vi "Create.vi"(7 "Direction":T1, 8 "error in (no error)":errorcluster, 9 "Custom Config Data":u8[](array[numeric]), 10 "Name":string, 11 "CIFTag in":refnum<class "CIF_NIChn_Fifo_Power.lvclass">) -> (0 "error out":errorcluster, 3 "CIFTag out":refnum<class "CIF_NIChn_Fifo_Power.lvclass">)   [LabVIEW 2021, in "CIF_NIChn_Fifo_Power.lvclass"]
uses:
  CIF_NIChn_Fifo_Power.lvclass
  CIF_NIChn_Fifo_Power.lvclass/CIF_NIChn_Fifo_Power.ctl
  CIFChannels/CIFChannels.lvclass
  CIFChannels/Typedef/Disconnect Behavior.ctl
  CIFChannels/Typedef/Channel State.ctl
  05c6e502-0377-480c-a15d-085597602460.vi
  c6f1aac1-fdda-4143-8087-f9e7d57e6170.vi
  D:/dev/Packages/Channel_Manager/src/CIF_NIChn/NIChn/CIF_NIChn.lvclass
  D:/dev/Packages/Channel_Manager/src/CIFChannels/CIFChannels.lvclass
  D:/dev/Packages/Channel_Manager/src/CIF_NIChn/FIFO_Power/CIF_NIChn_Fifo_Power.lvclass
  CIFChannels/Typedef/Direction.ctl
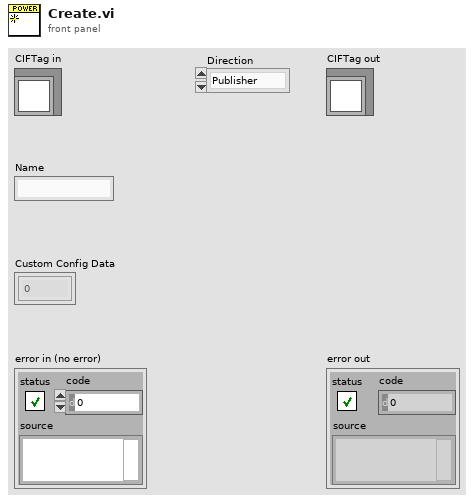
[diagram p1: front panel]
types:
  T1 = typedef "CIFChannels.lvclass/Direction.ctl" = enum16{"Publisher", "Subscriber"}
  T2 = typedef "CIFChannels.lvclass/Disconnect Behavior.ctl" = enum16{"Default value", "Last value", "Error with default"}
  T3 = typedef "CIFChannels.lvclass/Channel State.ctl" = enum16{"Creating", "Disconnected", "Connecting", "Connected", "Destroyed"}
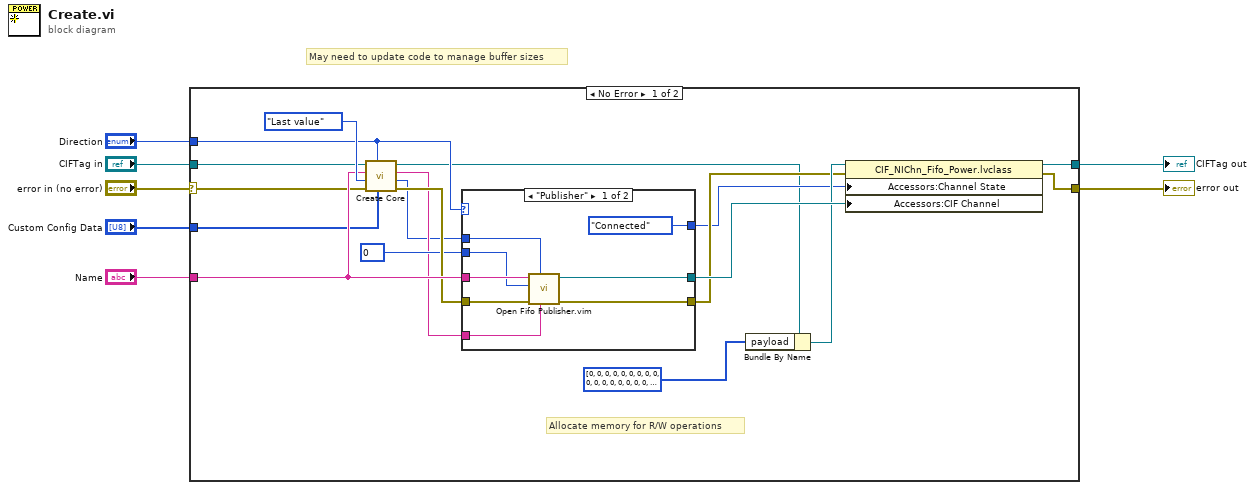
[diagram p0: block diagram]
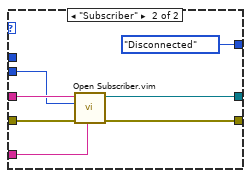
[diagram p2: hidden frame]
diagram:
  # "May need to update code to manage buffer sizes"
  n1 = case shown="No Error" "error in (no error)" {
    selector: "error in (no error)" -> [w9 w42]
    tunnel: [w8 w42] -> w6
    tunnel: [w19 w41] -> w4
    tunnel: "CIFTag in" -> [w10 w41]
    tunnel: "Name" -> [w24 _]
    tunnel: "Direction" -> [w18 _]
    tunnel: "Custom Config Data" -> [w12 _]
    frame No Error {
      # "Allocate memory for R/W operations"
      n2 = call "Create Core.vi"("Custom Config Data"=w12, "Direction"=w18, "error in (no error)"=w9, "Disconnect Behavior"=Disconnect_Behavior."Last value", "Name"=w24, "CIFChannels in"=w10) -> ("error out"=w23:errorcluster, "Depth"=w11:u64, "Channel Type"=w13:string, "CIFChannels out"=w16:refnum<class "CIF_NIChn_Fifo_Power.lvclass">)  [unwired: 2 in]
      n3 = case shown="\"Publisher\"" w18 {
        tunnel: w24 -> [w33 w39]
        tunnel: w23 -> [w32 w38]
        tunnel: [w28 w34] -> w22
        tunnel: [w29 w35] -> w20
        tunnel: w13 -> [w31 w37]
        tunnel: [Channel_State."Connected" ("Channel State") Channel_State."Disconnected" ("Channel State")] -> w17
        tunnel: u8 0 -> [w27 w36]
        tunnel: w11 -> [w26 _]
        frame "Publisher" {
          n4 = call "Open Fifo Publisher.vim"("Channel Type Description"=w31, "depth"=w26, "error in"=w32, "Input Type"=w27, "Channel Name"=w33) -> ("error out"=w29:errorcluster, "CIF Channel"=w28:refnum<k21>)  [unwired: 5 in]
        }
        frame "Subscriber" {
          n5 = call "Open Subscriber.vim"("Channel Type Description"=w37, "error in"=w38, "Input Type"=w36, "Channel Name"=w39) -> ("error out"=w35:errorcluster, "CIF Channel"=w34:refnum<k21>)  [unwired: 6 in]
        }
      }
      n6 = Bundle By Name(cluster=w16, "payload"=u8[] [0, 0, 0, 0, 0, 0, 0, 0, 0, 0, 0, 0, 0, 0, 0, 0, 0, 0, 0, 0, 0, 0, 0, 0, 0, 0, 0, 0, 0, 0, 0, 0, 0, 0, 0, 0, 0, 0, 0, 0, 0, 0, 0, 0, 0, 0, 0, 0, 0, 0, 0, 0, 0, 0, 0, 0, 0, 0, 0, 0, 0, 0, 0, 0, 0, 0, 0, 0, 0, 0, 0, 0, 0, 0, 0, 0, 0, 0, 0, 0, 0, 0, 0, 0, 0, 0, 0, 0, 0, 0, 0, 0, 0, 0, 0, 0, 0, 0, 0, 0, 0, 0, 0, 0, 0, 0, 0, 0, 0, 0, 0, 0, 0, 0, 0, 0, 0, 0, 0, 0, 0, 0, 0, 0, 0, 0, 0, 0, 0, 0, 0, 0, 0, 0, 0, 0, 0, 0, 0, 0, 0, 0, 0, 0, 0, 0, 0, 0, 0, 0, 0]) -> (w21:refnum<class "CIF_NIChn_Fifo_Power.lvclass">)
      n7 = property class="CIF_NIChn_Fifo_Power.lvclass"(reference=w21, error in=w20, "Accessors:Channel State"=w17, "Accessors:CIF Channel"=w22) -> (reference out=w19:refnum<class "CIF_NIChn_Fifo_Power.lvclass">, error out=w8:errorcluster)
    }
    frame Error {
    }
  }
  "error out" <- w6
  "CIFTag out" <- w4
